vi "price.vi"(8 "error in (no error)":errorcluster, 11 "VegBurger in":refnum<class "VegBurger.lvclass">) -> (0 "error out":errorcluster, 2 "price":dbl, 3 "VegBurger out":refnum<class "VegBurger.lvclass">)   [LabVIEW 2018, in "VegBurger.lvclass"]
uses:
  VegBurger.lvclass
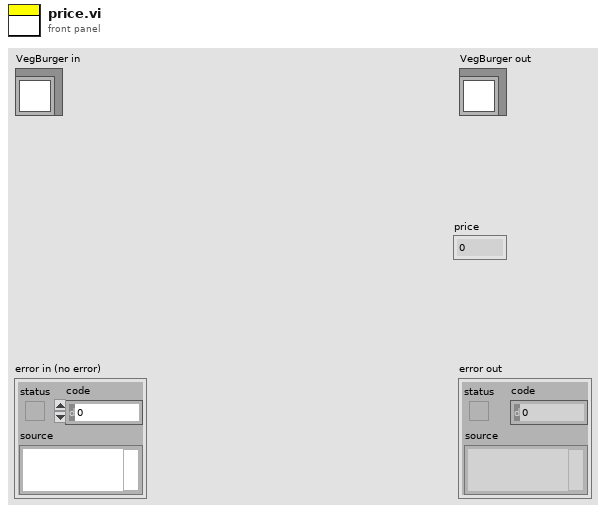
[diagram p1: front panel]
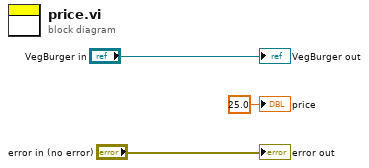
[diagram p0: block diagram]
diagram:
  "error out" <- "error in (no error)"
  "VegBurger out" <- "VegBurger in"
  "price" <- 25.0 ("price")
